vi "ControlWindowPos.vi"   [LabVIEW 2017]
uses:
  <vilib>/Utility/miscctls.llb/LVPoint32TypeDef.ctl
  Windows/System32/user32.dll
types:
  T1 = typedef "LVPoint32TypeDef.ctl" = cluster{"Horizontal":i32, "Vertical":i32}
  T2 = typedef "LVRectTypeDef.ctl" = cluster{"Left":i16, "Top":i16, "Right":i16, "Bottom":i16}
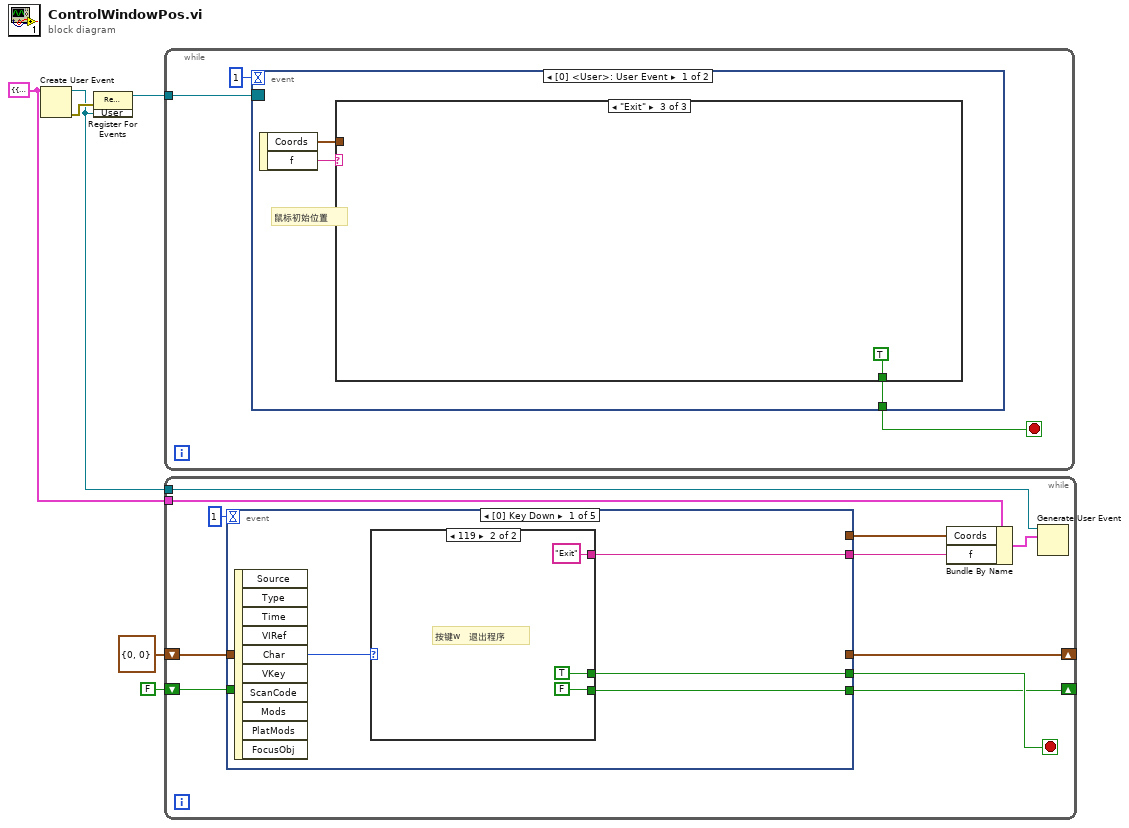
[diagram p0: block diagram]
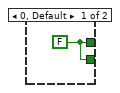
[diagram p2: hidden frame]
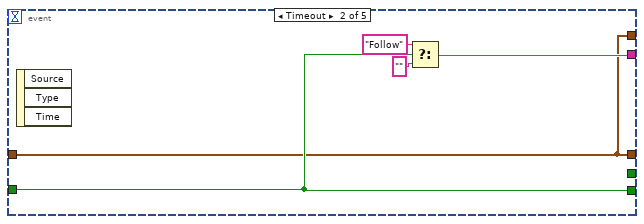
[diagram p3: hidden frame]
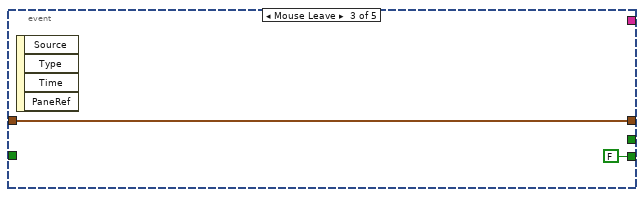
[diagram p4: hidden frame]
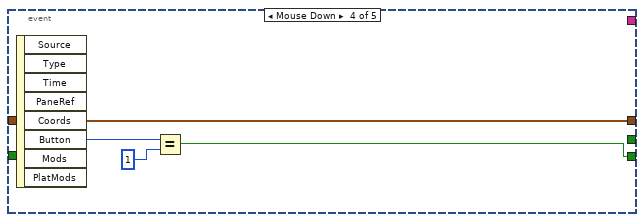
[diagram p5: hidden frame]
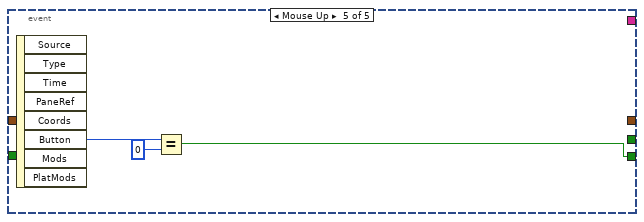
[diagram p6: hidden frame]
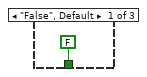
[diagram p7: hidden frame]
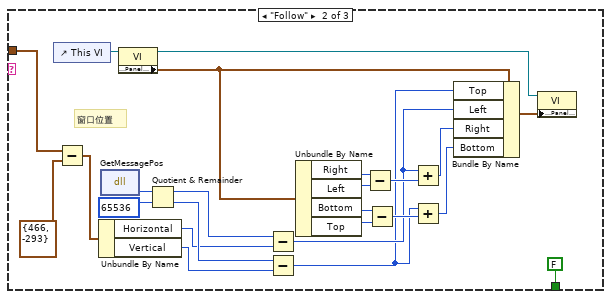
[diagram p8: hidden frame]
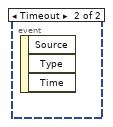
[diagram p9: hidden frame]
diagram:
  w1 = cluster{"Coords":T1, "f":string} {"Coords"={"Horizontal"=0, "Vertical"=0}, "f"=""} ("User")
  n1 = Create User Event(user event datatype=w1) -> (user event=w4:refnum<user-event>, error out=w6:errorcluster)  [unwired: 1 in]
  n2 = register-events(error in=w6, w4) -> (reference out=w5:refnum<event-registration>)  [unwired: 1 in, 1 out]
  n3 = while {
    tunnel: w5 -> [w8]
    stop <- w9 stop-if-true
    n4 = event shown="[0] <User>: User Event" {
      selector: w8 -> [_ _]
      dyn-events: _ -> [_ _]
      timeout: 1 -> [_ _]
      tunnel: [w12 _] -> w9
      event User Event {
        # "鼠标初始位置"
        n5 = event-data() -> ("Coords"=w10:T1, "f"=w11:string)  [unwired: 1 in]
        n6 = case shown="\"Exit\"" w11 {
          tunnel: [FALSE FALSE TRUE] -> w12
          tunnel: w10 -> [_ w18 _]
          frame "False", Default {
          }
          frame "Follow" {
            # "窗口位置"
            n7 = control-ref of="This VI"() -> (w35:refnum<vi>)
            n8 = Subtract(x=w18, y=T1 {"Horizontal"=466, "Vertical"=-293} ("Coords")) -> (x-y=w16:T1)
            n9 = Unbundle By Name(w16) -> ("Horizontal"=w15:i32, "Vertical"=w14:i32)
            n10 = dll-call lib="C:/Windows/System32/user32.dll" fn="GetMessagePos"() -> ("return type"=w37:i64)  [unwired: 3 in, 2 out]
            n11 = property class="VI"(reference=w35) -> (reference out=w33:refnum<vi>, "Front Panel.PanelBounds"=w34:T2)  [unwired: 1 in, 1 out]
            n12 = Quotient & Remainder(x=w37, y=i64 65536) -> (x-y*floor(x/y)=w19:i64, floor(x/y)=w22:i64)
            n13 = Subtract(x=w19, y=w15) -> (x-y=w21:i64)
            n14 = Subtract(x=w22, y=w14) -> (x-y=w20:i64)
            n15 = Unbundle By Name(w34) -> ("Right"=w32:i16, "Left"=w31:i16, "Bottom"=w30:i16, "Top"=w29:i16)
            n16 = Subtract(x=w32, y=w31) -> (x-y=w27:i16)
            n17 = Subtract(x=w30, y=w29) -> (x-y=w26:i16)
            n18 = Add(x=w21, y=w27) -> (x+y=w25:i64)
            n19 = Add(x=w20, y=w26) -> (x+y=w24:i64)
            n20 = Bundle By Name(cluster=w34, "Top"=w20, "Left"=w21, "Right"=w25, "Bottom"=w24) -> (w28:T2)
            n21 = property class="VI"(reference=w33, "Front Panel.PanelBounds"=w28) -> ()  [unwired: 1 in, 2 out]
          }
          frame "Exit" {
          }
        }
      }
      event Timeout {
        n22 = event-data() -> ()  [unwired: 1 in, 3 out]
      }
    }
  }
  n23 = while {
    tunnel: w4 -> [w48]
    shift-right: [w46] -> _
    shift-left: FALSE -> [w45]
    shift-right: [w44] -> _
    shift-left: T1 {"Horizontal"=0, "Vertical"=0} ("Coords") -> [w43]
    tunnel: w1 -> [w42]
    stop <- w49 stop-if-true
    n24 = event shown="[0] Key Down" {
      selector: _ -> [_ _ _ _ _]
      dyn-events: _ -> [_ _ _ _ _]
      timeout: 1 -> [_ _ _ _ _]
      tunnel: [w52 _ _ _ _] -> w49
      tunnel: [w51 w62 _ _ _] -> w39
      tunnel: [w50 w59 FALSE w66 w69] -> w46
      tunnel: w45 -> [_ w59 _ _ _]
      tunnel: [_ w58 w64 w65 _] -> w44
      tunnel: w43 -> [_ w58 w64 _ _]
      tunnel: [_ w58 _ _ _] -> w40
      event Key Down {
        n25 = event-data() -> ("Char"=w53:i16)  [unwired: 1 in, 9 out]
        n26 = case shown="119" w53 {
          tunnel: [_ "Exit" ("event data")] -> w51
          tunnel: [w54 TRUE] -> w52
          tunnel: [w54 FALSE] -> w50
          frame 0, Default {
            w54 = FALSE
          }
          frame 119 {
            # "按键w   退出程序"
          }
        }
      }
      event Timeout {
        n27 = event-data() -> ()  [unwired: 1 in, 3 out]
        n28 = Select(t="Follow" ("event data"), s=w59, f="") -> (s? t:f=w62:string)
      }
      event Mouse Leave {
        n29 = event-data() -> ()  [unwired: 1 in, 4 out]
      }
      event Mouse Down {
        n30 = event-data() -> ("Coords"=w65:T1, "Button"=w68:u16)  [unwired: 1 in, 6 out]
        n31 = Equal?(x=w68, y=u16 1) -> (x = y?=w66:bool)
      }
      event Mouse Up {
        n32 = event-data() -> ("Button"=w71:u16)  [unwired: 1 in, 7 out]
        n33 = Equal?(x=w71, y=u16 0) -> (x = y?=w69:bool)
      }
    }
    n34 = Bundle By Name(cluster=w42, "Coords"=w40, "f"=w39) -> (w41:cluster{"Coords":T1, "f":string})
    n35 = Generate User Event(user event=w48, event data cluster=w41) -> ()  [unwired: 2 in, 2 out]
  }
